vi "Convert Counts to Feet.vi"(5 "RevMotor/RevWheel":dbl=6.67 format="%#_13g", 7 "Wheel Diameter (in)":dbl=4.0 format="%#_13g", 10 "CPR (Ct/Rev mot)":dbl=2048.0, 11 "Counts":dbl) -> (3 "Ft":dbl)   [LabVIEW 2020, in "SwerveDrive_ACT.lvlib"]
uses:
  SwerveDrive_ACT.lvlib
panel:
  out "Inches":dbl
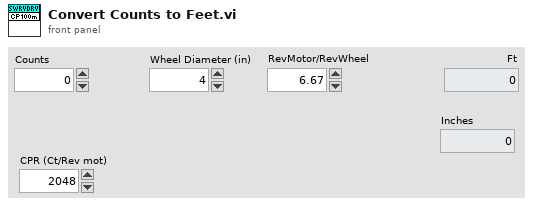
[diagram p1: front panel]
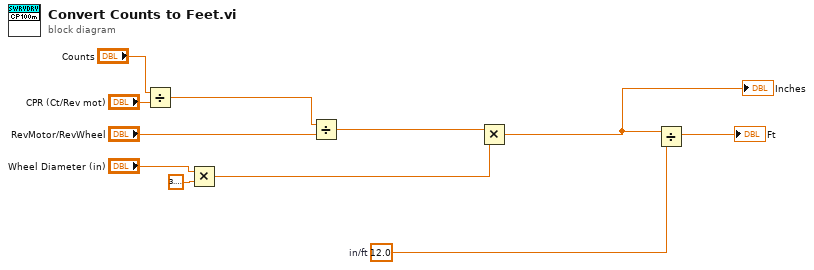
[diagram p0: block diagram]
diagram:
  w2 = 12.0  # in/ft
  n1 = Divide(x="Counts", y="CPR (Ct/Rev mot)") -> (x/y=w7:dbl)
  n2 = Multiply(x="Wheel Diameter (in)", y=3.141592653589793) -> (x*y=w4:dbl)
  n3 = Divide(x=w7, y="RevMotor/RevWheel") -> (x/y=w8:dbl)
  n4 = Multiply(x=w8, y=w4) -> (x*y=w1:dbl)
  "Inches" <- w1
  n5 = Divide(x=w1, y=w2) -> (x/y=→"Ft":dbl)
